vi "FTW-ProjectItemManager-Initialize.vi"(0 "Project Item Manager":refnum<class "FTW-ProjectItemManager.lvclass">, 5 "ProjectItem":refnum<vi>, 7 "Default Tag Values":refnum<class "FTW-Collection.lvclass">, 11 "error in":errorcluster) -> (4 "Project Item Manager out":refnum<class "FTW-ProjectItemManager.lvclass">, 15 "error out":errorcluster)   [LabVIEW 2012, in "FTW-ProjectItemManager.lvclass"]
uses:
  FTW-ProjectItemManager.lvclass
  Core/Collection/FTW-Collection.lvclass
  Core/Messaging/Messenger.Actor/FTW-Messenger-Actor.lvclass
  FTW-ProjectItemManager.lvclass/FTW-ProjectItemManager.ctl
panel:
  # "Inputs"
  # "Outputs"
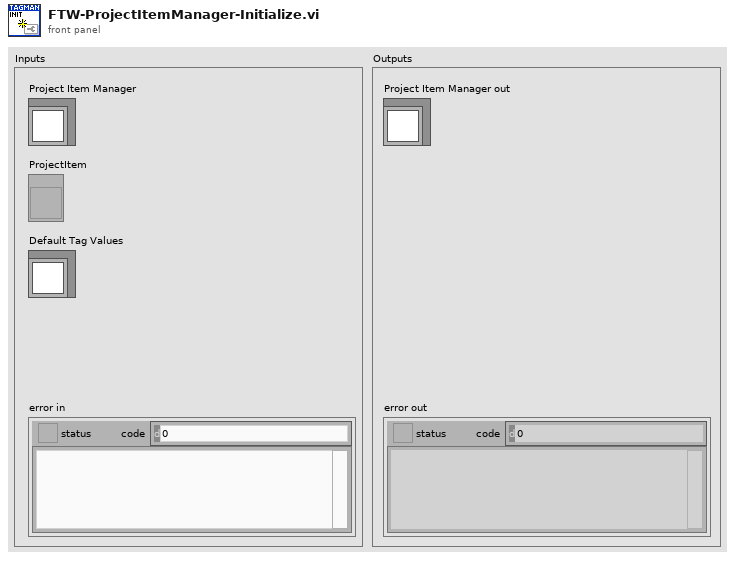
[diagram p1: front panel]
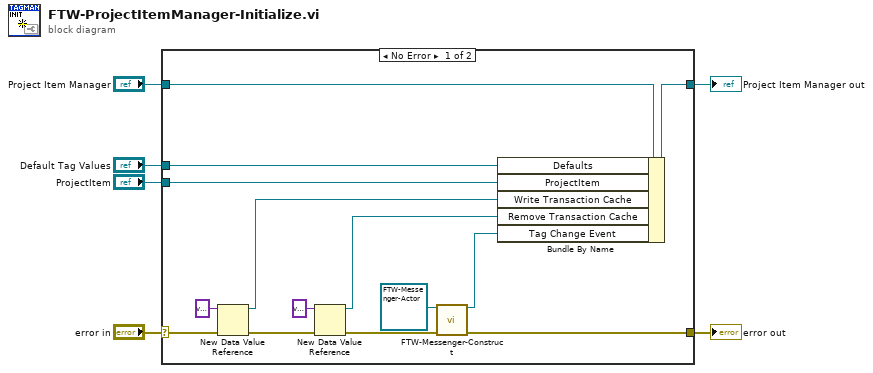
[diagram p0: block diagram]
diagram:
  n1 = case shown="No Error" "error in" {
    selector: "error in" -> [w7 w22]
    tunnel: [w11 w22] -> w6
    tunnel: [w19 w21] -> w5
    tunnel: "Project Item Manager" -> [w20 w21]
    tunnel: "Default Tag Values" -> [w9 _]
    tunnel: "ProjectItem" -> [w8 _]
    frame No Error {
      n2 = New Data Value Reference(data value=variant, error in=w7) -> (data value reference=w17:refnum<data-value>, error out=w14:errorcluster)
      n3 = New Data Value Reference(data value=variant, error in=w14) -> (data value reference=w15:refnum<data-value>, error out=w13:errorcluster)
      n4 = call-dynamic "FTW-Messenger-Construct.vi"("Messenger Type"=refnum<class "FTW-Messenger-Actor.lvclass"> refnum, "error in"=w13) -> ("Actor Messenger"=w12:refnum<class "FTW-Messenger-Actor.lvclass">, "error out"=w11:errorcluster)  [unwired: 12 in]
      n5 = Bundle By Name(cluster=w20, "Defaults"=w9, "ProjectItem"=w8, "Write Transaction Cache"=w17, "Remove Transaction Cache"=w15, "Tag Change Event"=w12) -> (w19:refnum<class "FTW-ProjectItemManager.lvclass">)
    }
    frame Error {
    }
  }
  "error out" <- w6
  "Project Item Manager out" <- w5
